vi "Replace File.vi"(8 "error in (no error)":errorcluster, 11 "Configuration File in":refnum<class "Configuration File.lvclass">) -> (0 "error out":errorcluster, 3 "Configuration File out":refnum<class "Configuration File.lvclass">)   [LabVIEW 2019, in "Configuration File.lvlib" / "Configuration File.lvclass"]
doc: "DO NOT USE IN THE ROBOT'S CODE. EVER.\n\nThis VI will delete the currently open config file and create a new one with the same name. Use this when you need to recreate the configuration file."
uses:
  Configuration File.lvclass
  Configuration File.lvclass/Configuration File.ctl
  <vilib>/Utility/config.llb/NI_LVConfig.lvlib
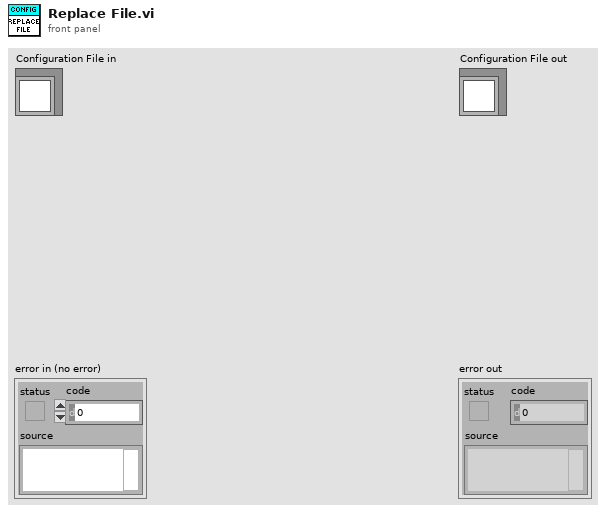
[diagram p1: front panel]
types:
  T1 = typedef "NI_LVConfig.lvlib/Config Data RefNum.ctl" = refnum<k1>
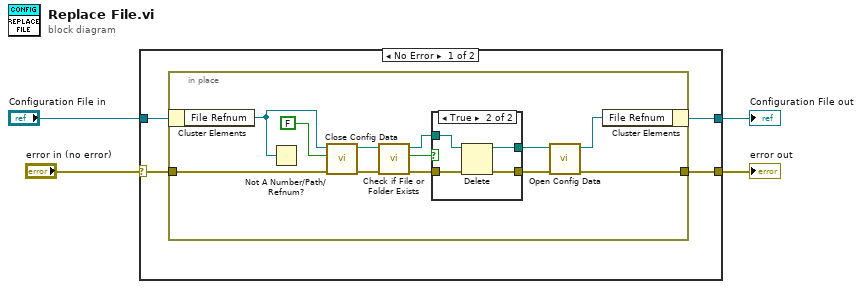
[diagram p0: block diagram]
diagram:
  n1 = case shown="No Error" "error in (no error)" {
    selector: "error in (no error)" -> [w6 w28]
    tunnel: [w5 w28] -> w3
    tunnel: [w8 w27] -> w1
    tunnel: "Configuration File in" -> [w7 w27]
    frame No Error {
      n2 = in-place {
        in-place-border: w6 -> [w19]
        in-place-border: [w18] -> w5
        n3 = in-place-cluster #1(w7) -> ("File Refnum"=w17:T1)
        n4 = Not A Number/Path/Refnum?(number/path/refnum=w17) -> ()  [unwired: 1 out]
        n5 = call <vilib>:"Close Config Data.vi"("error in (no error)"=w19, "write file if changed (T)"=FALSE, "refnum"=w17) -> ("error out"=w11:errorcluster, "file path"=w16:path)  [unwired: 7 in]
        n6 = call <vilib>:"Check if File or Folder Exists.vi"("error in (no error)"=w11, "path"=w16) -> ("error out"=w12:errorcluster, "file or folder exists?"=w10:bool, "dup path"=w15:path)  [unwired: 7 in]
        n7 = case shown="True" w10 {
          tunnel: w15 -> [w22 w26]
          tunnel: [w22 w25] -> w14
          tunnel: [w21 w24] -> w13
          tunnel: w12 -> [w21 w23]
          frame False {
          }
          frame True {
            n8 = Delete(path (use dialog)=w26, error in=w23) -> (deleted path=w25:path, error out=w24:errorcluster)  [unwired: 3 in, 1 out]
          }
        }
        n9 = call <vilib>:"Open Config Data.vi"("error in (no error)"=w13, "configuration file path"=w14) -> ("error out"=w18:errorcluster, "refnum"=w20:T1)  [unwired: 7 in, 1 out]
        n10 = in-place-cluster #1("File Refnum"=w20) -> (w8:refnum<class "Configuration File.lvclass">)
      }
    }
    frame Error {
    }
  }
  "error out" <- w3
  "Configuration File out" <- w1
